vi "Initialize Library.vi"(8 "error in":errorcluster) -> (0 "error out":errorcluster, 2 "modules found":i32)   [LabVIEW 2020, in "AIM ARINC 429 Hardware API.lvlib"]
uses:
  AIM ARINC 429 Hardware API.lvlib
  <instrlib>/AIM GmbH/ARINC-429/AIM429LV.lvlib
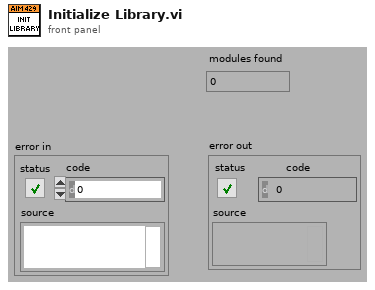
[diagram p1: front panel]
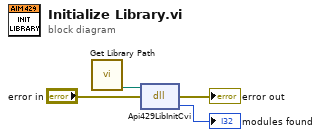
[diagram p0: block diagram]
diagram:
  n1 = call <instrlib>:"Get Library Path.vi"() -> ("GlobalDLLPath"=w3:path)  [unwired: 11 in]
  n2 = dll-call lib="api_civ.9.dll" fn="Api429LibInitCvi"(path in=w3, error in="error in") -> (error out=→"error out":errorcluster, "modules found"=→"modules found":i32)  [unwired: 1 in, 1 out]
